vi "Clock.vi"() -> ()   [LabVIEW 2018]
panel:
  in  "Boolean":bool
  out "Get Date/Time in Seconds Control":timestamp
  out "Format Date/Time String Control":string
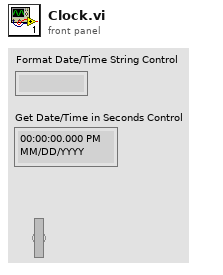
[diagram p1: front panel]
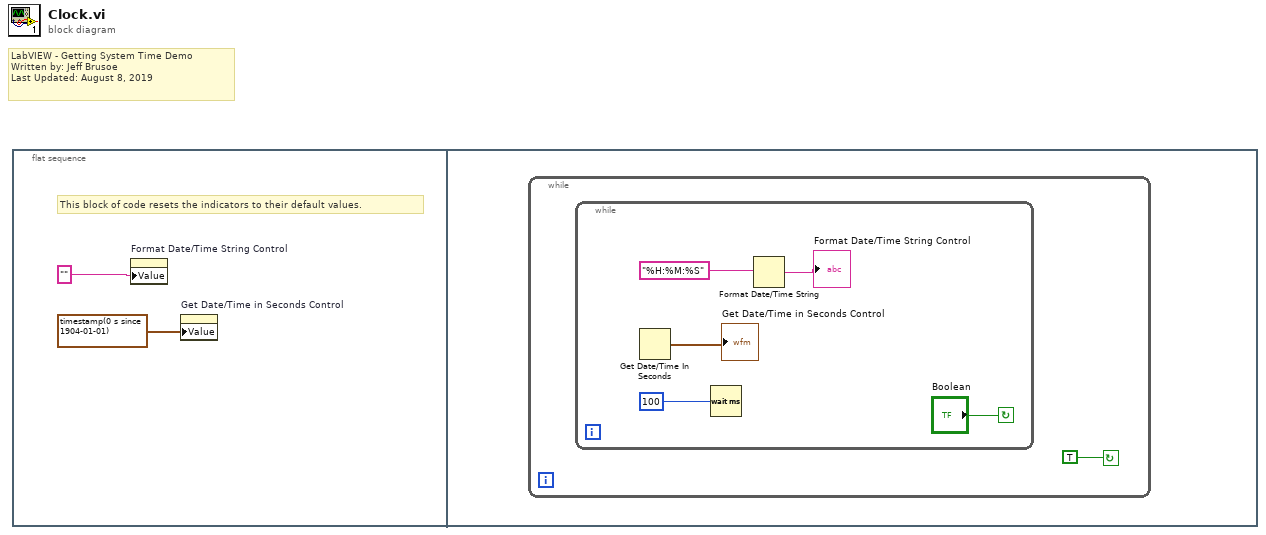
[diagram p0: block diagram]
diagram:
  # "LabVIEW - Getting System Time Demo\nWritten by: Jeff Brusoe\nLast Updated: August 8, 2019"
  n1 = flat-sequence {
    frame #0 {
      # "This block of code resets the indicators to their default values."
      n2 = property on="Format Date/Time String Control" class="Str"("Value"="") -> ()  [unwired: 2 in, 2 out]
      n3 = property on="Get Date/Time in Seconds Control" class="AbsTime (strict)"("Value"=timestamp(0 s since 1904-01-01)) -> ()  [unwired: 2 in, 2 out]
    }
    frame #1 {
      n4 = while {
        stop <- TRUE continue-if-true
        n5 = while {
          stop <- "Boolean" continue-if-true
          n6 = Get Date/Time In Seconds() -> (seconds since 1Jan1904=→"Get Date/Time in Seconds Control":timestamp)
          n7 = Wait (ms)(milliseconds to wait=100) -> ()  [unwired: 1 out]
          n8 = Format Date/Time String(time format string (%c)="%H:%M:%S") -> (date/time string=→"Format Date/Time String Control":string)  [unwired: 2 in]
        }
      }
    }
  }
